vi "Numeric Array To String.vi"   [LabVIEW 2019, in "Agilent 3352X Series.lvlib"]
doc: "Phase a numeric array to a serial string seperated by specifc characters."
uses:
  Agilent 3352X Series.lvlib
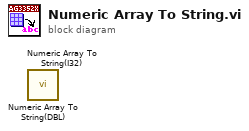
[diagram p0: block diagram]
diagram:
  n1 = call "Numeric Array To String(DBL).vi"() -> ()  [unwired: 11 in, 1 out]
  n2 = call "Numeric Array To String(I32).vi"() -> ()  [unwired: 11 in, 1 out]
